vi "Filter Outbound Message.vi"(7 "Message":refnum<class "Message.lvclass">, 10 "Receiver Info":T1, 11 "Pub Sub Message Channel in":refnum<class "Pub Sub Message Channel.lvclass">) -> (3 "Drop Message":bool)   [LabVIEW 2020, in "Actor Pub Sub Channels.lvlib" / "Pub Sub Message Channel.lvclass"]
uses:
  Pub Sub Message Channel.lvclass
  <vilib>/ActorFramework/Message/Message.lvclass
  Pub Sub Message Channel.lvclass/Pub Sub Message Channel.ctl
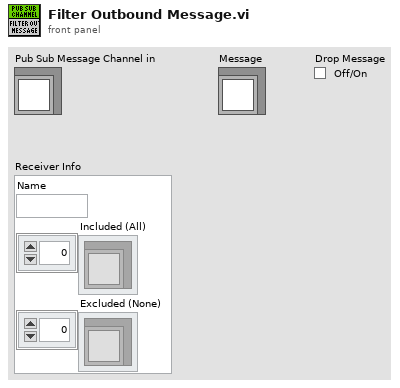
[diagram p1: front panel]
types:
  T1 = cluster{"Name":string, "Included (All)":refnum<class>[], "Excluded (None)":refnum<class>[]}
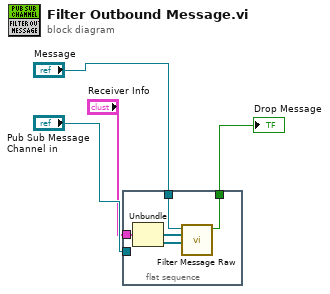
[diagram p0: block diagram]
diagram:
  n1 = flat-sequence {
    tunnel: "Receiver Info" -> [w9]
    tunnel: "Pub Sub Message Channel in" -> [_]
    tunnel: "Message" -> [w6]
    tunnel: [w5] -> w4
    frame #0 {
      n2 = Unbundle(w9) -> ("Included (All)"=w7:refnum<class>[], "Excluded (None)"=w8:refnum<class>[])  [unwired: 1 out]
      n3 = call "Filter Message Raw.vi"("Excluded Message Types"=w8, "Included Message Types"=w7, "Message in"=w6) -> ("Checkbox"=w5:bool)  [unwired: 8 in]
    }
  }
  "Drop Message" <- w4
